vi "testRegTelServersAandB.vi"(8 "error in (no error)":errorcluster) -> (0 "error out":errorcluster)   [LabVIEW 2018]
uses:
  src/FactoryTcpServer/FactoryTcpServer.lvclass
  src/TcpServer/TcpServer.lvclass/TcpServer.ctl
  src/TcpServerBase/TcpServerBase.lvclass/TcpServerBase.ctl
  src/TcpServerTel/TcpServerTel.lvclass
  home/pcortes/Documents/github/ts_labview_tcp_json/src/TcpServerBase/TcpServerBase.lvclass
  <vilib>/addons/_JKI Toolkits/Caraya/classes/Assert/Assert Equal Value_Variant.vi
  <vilib>/addons/_JKI Toolkits/Caraya/classes/Test/Test.lvclass
  <vilib>/addons/_JKI Toolkits/Caraya/classes/Assert/Assert.lvclass
  src/TcpServerBase/TcpServerBase.lvclass
  src/TcpServer/TcpServer.lvclass
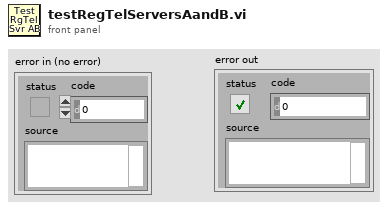
[diagram p1: front panel]
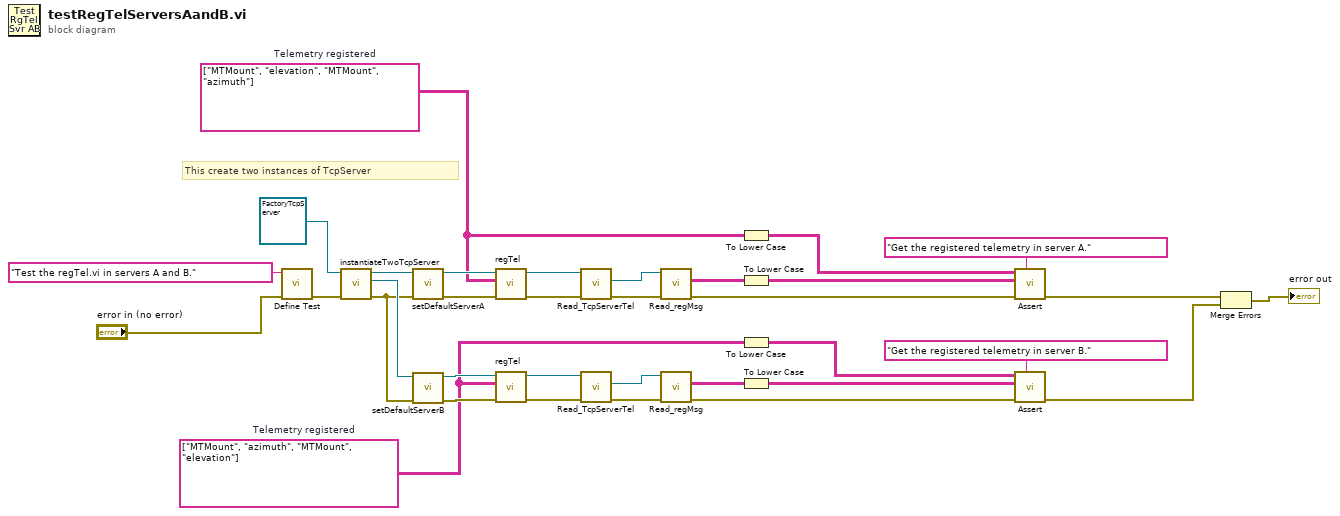
[diagram p0: block diagram]
diagram:
  w7 = string[][] [["MTMount", "azimuth"], ["MTMount", "elevation"]]  # Telemetry registered
  w18 = string[][] [["MTMount", "elevation"], ["MTMount", "azimuth"]]  # Telemetry registered
  # "This create two instances of TcpServer"
  n1 = call <vilib>:"Define Test.vi"("error in (no error)"="error in (no error)", "Label (VI Title)"="Test the regTel.vi in servers A and B.") -> ("error out"=w4:errorcluster)  [unwired: 9 in]
  n2 = call "instantiateTwoTcpServer.vi"("error in (no error)"=w4, "FactoryTcpServer in"=refnum<class "FactoryTcpServer.lvclass"> refnum) -> ("error out"=w1:errorcluster, "TcpServer 2 out"=w2:refnum<class "TcpServer.lvclass">, "TcpServer 1 out"=w3:refnum<class "TcpServer.lvclass">)  [unwired: 7 in]
  n3 = call "setDefaultServerA.vi"("error in (no error)"=w1, "TcpServer.lvclass"=w3) -> ("error out"=w20:errorcluster, "tcpServer out"=w19:refnum<class "TcpServer.lvclass">)  [unwired: 8 in]
  n4 = call "setDefaultServerB.vi"("error in (no error)"=w1, "TcpServer.lvclass"=w2) -> ("error out"=w11:errorcluster, "tcpServer out"=w10:refnum<class "TcpServer.lvclass">)  [unwired: 8 in]
  n5 = call "regTel.vi"("error in (no error)"=w20, "telReg"=w18, "tcpServer in"=w19) -> ("error out"=w22:errorcluster, "tcpServer out"=w23:refnum<class "TcpServer.lvclass">)  [unwired: 7 in]
  n6 = call "regTel.vi"("error in (no error)"=w11, "telReg"=w7, "tcpServer in"=w10) -> ("error out"=w13:errorcluster, "tcpServer out"=w12:refnum<class "TcpServer.lvclass">)  [unwired: 7 in]
  n7 = call "Read_TcpServerTel.vi"("error in (no error)"=w22, "TcpServer in"=w23) -> ("error out"=w6:errorcluster, "TcpServerTel.lvclass"=w21:refnum<class "TcpServerTel.lvclass">)  [unwired: 7 in, 1 out]
  n8 = call "Read_TcpServerTel.vi"("error in (no error)"=w13, "TcpServer in"=w12) -> ("error out"=w15:errorcluster, "TcpServerTel.lvclass"=w14:refnum<class "TcpServerTel.lvclass">)  [unwired: 7 in, 1 out]
  n9 = call "Read_regMsg.vi"("error in (no error)"=w6, "TcpServerBase in"=w21) -> ("error out"=w16:errorcluster, "regMsg"=w17:string[][])  [unwired: 7 in, 1 out]
  n10 = call "Read_regMsg.vi"("error in (no error)"=w15, "TcpServerBase in"=w14) -> ("error out"=w9:errorcluster, "regMsg"=w8:string[][])  [unwired: 7 in, 1 out]
  n11 = To Lower Case(string=w18) -> (all lower case string=w27:string[][])
  n12 = To Lower Case(string=w17) -> (all lower case string=w26:string[][])
  n13 = To Lower Case(string=w7) -> (all lower case string=w25:string[][])
  n14 = To Lower Case(string=w8) -> (all lower case string=w24:string[][])
  n15 = call-poly <vilib>:"Assert.vi"("Label"="Get the registered telemetry in server A.", "error in (no error)"=w16, "Y"=w26, "X"=w27) -> ("error out"=w32:errorcluster)  [unwired: 7 in]
  n16 = call-poly <vilib>:"Assert.vi"("Label"="Get the registered telemetry in server B.", "error in (no error)"=w9, "Y"=w24, "X"=w25) -> ("error out"=w28:errorcluster)  [unwired: 7 in]
  n17 = Merge Errors(w32, w28) -> (→"error out":errorcluster)
